vi "SystemController.SetImage.vi"(8 "error in (no error)":errorcluster, 10 "Image":T1, 11 "SystemController":refnum<class "SystemController.lvclass">) -> (0 "error out":errorcluster, 3 "SystemController out":refnum<class "SystemController.lvclass">)   [LabVIEW 2017, in "SystemController.lvclass"]
doc: "---------------------------------------------------------------\nJKI State Machine Objects™\nhttp://jki.net/state-machine-objects/\nCopyright (C) 2005-2015, JKI <info@jki.net>\nALL RIGHTS RESERVEDJKI State Machine Objects (SMO) 1.0.0.5\nJKI - JKI\nCopyright (c) 2016, JKI"
uses:
  SystemController.lvclass
  <vilib>/vision/Image Controls.llb/IMAQ Image.ctl
  SystemController.lvclass/SystemController.ctl
panel:
  # "For instructions on how to use the JKI State Machine Objects, examples and video tutorials, visit:\nhttp://jki.net/state-machine-objects/\n\nJKI State Machine Objects™\nhttp://jki.net/state-machine-objects/\nCopyright (C) 2005-2015, JKI <info@jki.net>\nALL RIGHTS RESERVED"
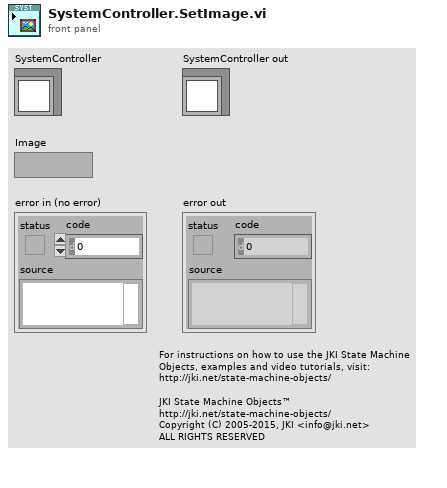
[diagram p1: front panel]
types:
  T1 = typedef "IMAQ Image.ctl" = refnum<image>
  T2 = typedef "SystemController.lvclass/PrivateData--Ref.ctl" = refnum<data-value>
  T3 = typedef "SystemController.lvclass/PrivateData--Cluster.ctl" = cluster{"Configuration":T4, "Dependencies":T8, "Public Events":T9, "Processed Image Buffer":T1[]}
  T4 = typedef "SystemController.lvclass/Configuration--Cluster.ctl" = cluster{"Camera":T5, "Find Eyes":bool, "Acquisition Rate (ms)":i32, "Image Buffer Length":i32}
  T5 = typedef "SystemController.lvclass/CameraConfig--Cluster.ctl" = cluster{"Simulate Camera":bool, "IMAQ Camera":T6, "Simulated Camera Image":path}
  T6 = typedef "Camera_IMAQdx.lvclass/Configuration--Cluster.ctl" = cluster{"Camera Interface Name":string, "Number of Buffers":u32, "Image Name":string, "Image Type":T7}
  T7 = typedef "Image Type" = u32
  T8 = typedef "SystemController.lvclass/Dependencies--Cluster.ctl" = cluster{"Camera":refnum<class "Camera.lvclass">, "ImageFacialDetection":refnum<class "ImageFacialDetection.lvclass">}
  T9 = typedef "SystemController.lvclass/PublicEvents--Cluster.ctl" = cluster{"UIClosed":refnum<user-event>}
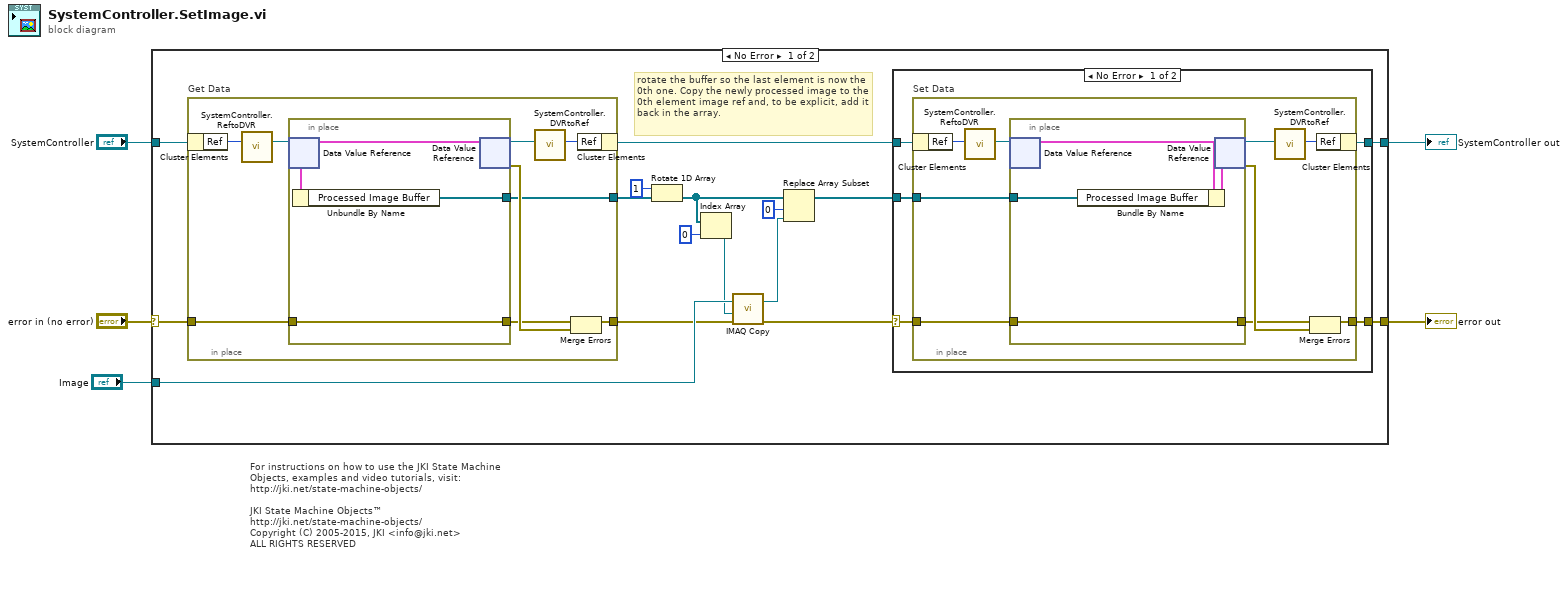
[diagram p0: block diagram]
diagram:
  # "For instructions on how to use the JKI State Machine Objects, examples and video tutorials, visit:\nhttp://jki.net/state-machine-objects/\n\nJKI State Machine Objects™\nhttp://jki.net/state-machine-objects/\nCopyright (C) 2005-2015, JKI <info@jki.net>\nALL RIGHTS RESERVED"
  n1 = case shown="No Error" "error in (no error)" {
    selector: "error in (no error)" -> [w20 w54]
    tunnel: "SystemController" -> [w21 w55]
    tunnel: [w18 w54] -> w4
    tunnel: [w17 w55] -> w3
    tunnel: "Image" -> [w13 _]
    frame No Error {
      # "rotate the buffer so the last element is now the 0th one. Copy the newly processed image to the 0th element image ref and, to be explicit, add it back in the array."
      n2 = in-place "Get Data" {
        in-place-border: w20 -> [w50]
        in-place-border: [w47] -> w7
        in-place-border: [w46] -> w16
        n3 = in-place-cluster #1(w21) -> ("Ref"=w45:u32)
        n4 = call "SystemController.ReftoDVR.vi"("Ref"=w45) -> ("Ref"=w44:T2)  [unwired: 10 in]
        n5 = in-place {
          in-place-border: w50 -> [w52]
          in-place-border: [w52] -> w48
          in-place-border: [w51] -> w46
          n6 = in-place-dvr #2(w44) -> (w53:T3)  [unwired: 1 out]
          n7 = Unbundle By Name(w53) -> ("Processed Image Buffer"=w51:T1[])
          n8 = in-place-dvr #2(w53) -> (w43:T2, w49:errorcluster)
        }
        n9 = call "SystemController.DVRtoRef.vi"("Ref"=w43) -> ("Ref"=w42:u32)  [unwired: 10 in]
        n10 = Merge Errors(w48, w49) -> (w47:errorcluster)
        n11 = in-place-cluster #1("Ref"=w42) -> (w19:refnum<class "SystemController.lvclass">)
      }
      n12 = Rotate 1D Array(1:w16, 2:1 ("n")) -> (0:w11:T1[])
      n13 = Index Array(array=w11, index=0) -> (element=w12:T1)
      n14 = call "IMAQ Copy"("error in (no error)"=w7, "Image Dst"=w12, "Image Src"=w13) -> ("error out"=w6:errorcluster, "Image Dst Out"=w8:T1)  [unwired: 3 in]
      n15 = Replace Array Subset(array=w11, new element=w8, index=0) -> (w10:T1[])
      n16 = case shown="No Error" w6 {
        selector: w6 -> [w22 w40]
        tunnel: w19 -> [w26 w41]
        tunnel: [w25 w40] -> w18
        tunnel: [w24 w41] -> w17
        tunnel: w10 -> [w23 _]
        frame No Error {
          n17 = in-place "Set Data" {
            in-place-border: w22 -> [w35]
            in-place-border: [w32] -> w25
            in-place-border: w23 -> [w31]
            n18 = in-place-cluster #3(w26) -> ("Ref"=w30:u32)
            n19 = call "SystemController.ReftoDVR.vi"("Ref"=w30) -> ("Ref"=w29:T2)  [unwired: 10 in]
            n20 = in-place {
              in-place-border: w35 -> [w38]
              in-place-border: [w38] -> w33
              in-place-border: w31 -> [w36]
              n21 = in-place-dvr #4(w29) -> (w39:T3)  [unwired: 1 out]
              n22 = Bundle By Name(cluster=w39, "Processed Image Buffer"=w36) -> (w37:T3)
              n23 = in-place-dvr #4(w37) -> (w28:T2, w34:errorcluster)
            }
            n24 = call "SystemController.DVRtoRef.vi"("Ref"=w28) -> ("Ref"=w27:u32)  [unwired: 10 in]
            n25 = Merge Errors(w33, w34) -> (w32:errorcluster)
            n26 = in-place-cluster #3("Ref"=w27) -> (w24:refnum<class "SystemController.lvclass">)
          }
        }
        frame Error {
          # "Do not write back on error"
        }
      }
    }
    frame Error {
    }
  }
  "error out" <- w4
  "SystemController out" <- w3
